vi "go2zero.vi"() -> ()   [LabVIEW 2015]
panel:
  in  "Motor":u16(ring) items=["X", "Y", "Z", "Gluer", "Spint"]
  out "command":string
  out "output":string
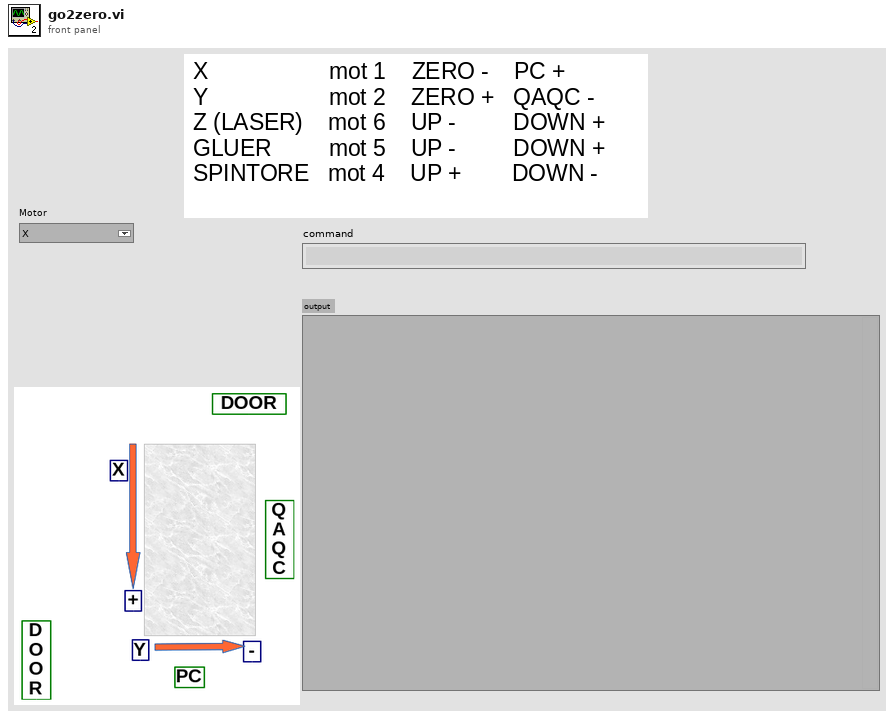
[diagram p1: front panel]
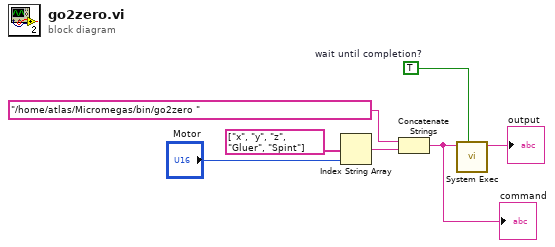
[diagram p0: block diagram]
diagram:
  w7 = TRUE  # wait until completion?
  n1 = Index String Array(1:"Motor", 2:string[] ["x", "y", "z", "Gluer", "Spint"] ("string array")) -> (0:w1:string)  [unwired: 1 in]
  n2 = Concatenate Strings("/home/atlas/Micromegas/bin/go2zero " ("string"), w1) -> (w5:string)
  "command" <- w5
  n3 = call <vilib>:"System Exec.vi"("wait until completion? (T)"=w7, "command line"=w5) -> ("standard output"=→"output":string)  [unwired: 6 in, 3 out]
